vi "Draw Robot.vi"(7 "Gyro":dbl=-0.11, 8 "Starting Location":u16(ring)=2 items=["Left", "Center", "Right"], 10 "XY":cluster{"X":dbl, "Y":dbl}) -> (2 "Graph 2":cluster{cluster{"X":dbl, "Y":dbl}[]}[](graph)=[{[{"X"=44.0, "Y"=76.0}, {"X"=44.0, "Y"=76.0}]}, {[{"X"=30.03458329904793, "Y"=57.973155118857626}, {"X"=30.03458329904793, "Y"=57.973155118857626}]}, {[{"X"=29.965468303127132, "Y"=93.97308877320398}, {"X"=29.965468303127132, "Y"=93.97308877320398}]}, {[{"X"=57.96541670095207, "Y"=94.02684488114238}, {"X"=57.96541670095207, "Y"=94.02684488114238}]}, {[{"X"=58.03453169687287, "Y"=58.026911226796024}, {"X"=58.03453169687287, "Y"=58.026911226796024}]}, {[{"X"=43.942404170066, "Y"=105.9999447119553}, {"X"=43.942404170066, "Y"=105.9999447119553}]}])   [LabVIEW 2018]
panel:
  in  "Robot Lenght":dbl=44.0
  in  "Robot Width":dbl=28.0
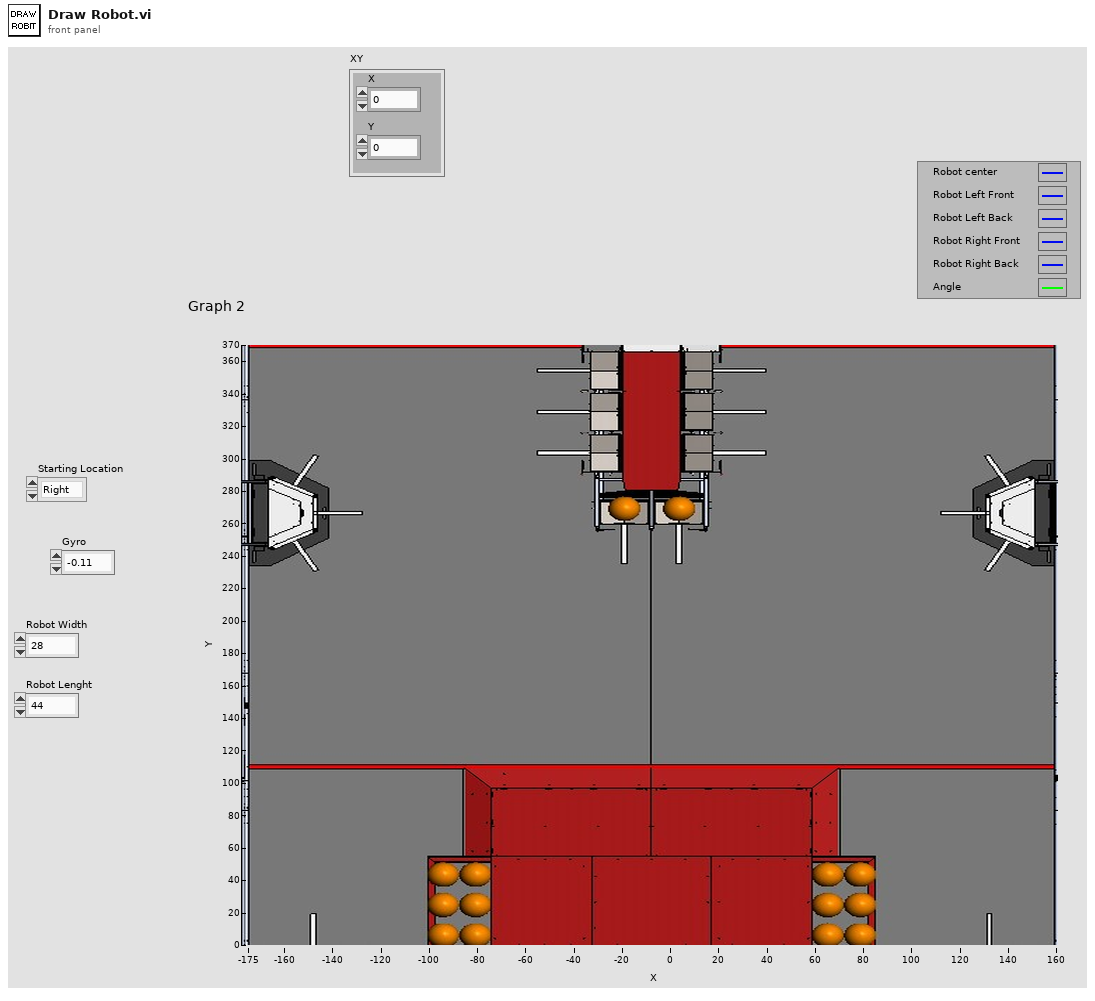
[diagram p1: front panel]
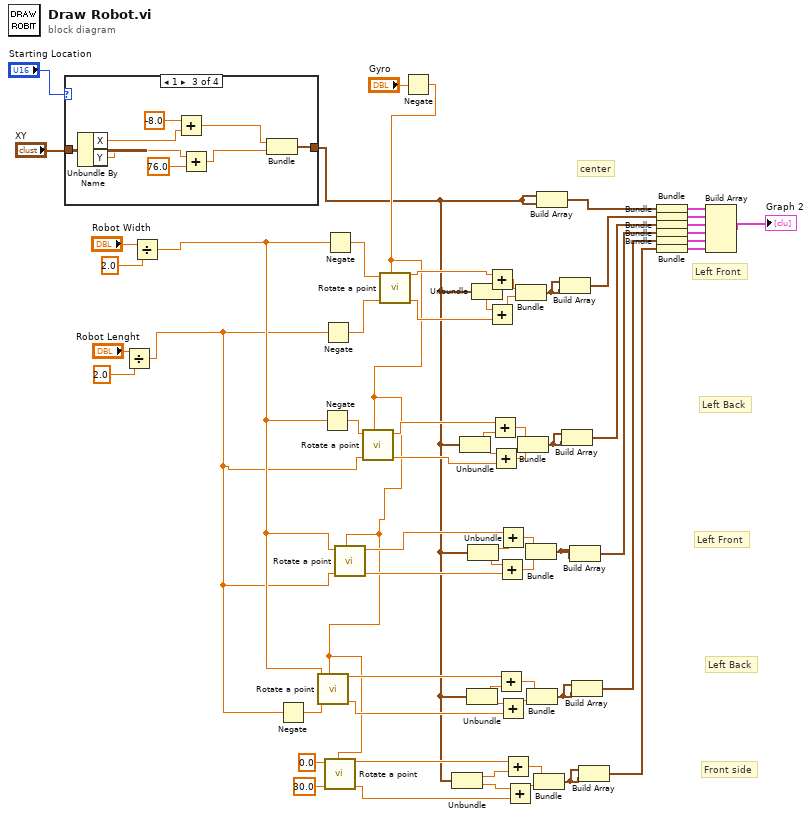
[diagram p0: block diagram]
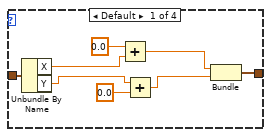
[diagram p2: hidden frame]
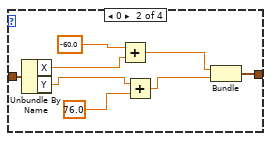
[diagram p3: hidden frame]
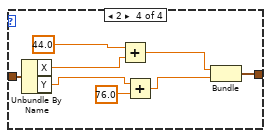
[diagram p4: hidden frame]
diagram:
  # "center"
  # "Front side"
  # "Left Back"
  # "Left Front"
  # "Left Back"
  # "Left Front"
  n1 = case shown="1" "Starting Location" {
    tunnel: "XY" -> [w73 w81 w89 w97]
    tunnel: [w72 w80 w88 w96] -> w2
    frame Default {
      n2 = Unbundle By Name(w73) -> ("X"=w71:dbl, "Y"=w69:dbl)
      n3 = Add(x=0.0, y=w71) -> (x+y=w70:dbl)
      n4 = Add(x=w69, y=0.0) -> (x+y=w68:dbl)
      n5 = Bundle(w70, w68) -> (w72:cluster{dbl, dbl})  [unwired: 1 in]
    }
    frame 0 {
      n6 = Unbundle By Name(w81) -> ("X"=w79:dbl, "Y"=w77:dbl)
      n7 = Add(x=-60.0, y=w79) -> (x+y=w78:dbl)
      n8 = Add(x=w77, y=76.0) -> (x+y=w76:dbl)
      n9 = Bundle(w78, w76) -> (w80:cluster{dbl, dbl})  [unwired: 1 in]
    }
    frame 1 {
      n10 = Unbundle By Name(w89) -> ("X"=w87:dbl, "Y"=w85:dbl)
      n11 = Add(x=-8.0, y=w87) -> (x+y=w86:dbl)
      n12 = Add(x=w85, y=76.0) -> (x+y=w84:dbl)
      n13 = Bundle(w86, w84) -> (w88:cluster{dbl, dbl})  [unwired: 1 in]
    }
    frame 2 {
      n14 = Unbundle By Name(w97) -> ("X"=w95:dbl, "Y"=w93:dbl)
      n15 = Add(x=44.0, y=w95) -> (x+y=w94:dbl)
      n16 = Add(x=w93, y=76.0) -> (x+y=w92:dbl)
      n17 = Bundle(w94, w92) -> (w96:cluster{dbl, dbl})  [unwired: 1 in]
    }
  }
  n18 = Divide(x="Robot Lenght", y=2.0) -> (x/y=w45:dbl)
  n19 = Divide(x="Robot Width", y=2.0) -> (x/y=w46:dbl)
  n20 = Negate(x=w45) -> (-x=w50:dbl)
  n21 = Negate(x=w46) -> (-x=w47:dbl)
  n22 = Negate(x=w45) -> (-x=w48:dbl)
  n23 = Negate(x=w46) -> (-x=w49:dbl)
  n24 = Negate(x="Gyro") -> (-x=w4:dbl)
  n25 = call "Rotate a point.vi"("Gyro"=w4, "Y"=w50, "X"=w46) -> ("Y'"=w21:dbl, "X'"=w22:dbl)  [unwired: 7 in]
  n26 = call "Rotate a point.vi"("Gyro"=w4, "Y"=30.0, "X"=0.0) -> ("Y'"=w16:dbl, "X'"=w15:dbl)  [unwired: 7 in]
  n27 = call "Rotate a point.vi"("Gyro"=w4, "Y"=w45, "X"=w46) -> ("Y'"=w23:dbl, "X'"=w24:dbl)  [unwired: 7 in]
  n28 = call "Rotate a point.vi"("Gyro"=w4, "Y"=w45, "X"=w47) -> ("Y'"=w33:dbl, "X'"=w34:dbl)  [unwired: 7 in]
  n29 = call "Rotate a point.vi"("Gyro"=w4, "Y"=w48, "X"=w49) -> ("Y'"=w39:dbl, "X'"=w40:dbl)  [unwired: 7 in]
  n30 = Unbundle(w2) -> (w9:dbl, w8:dbl)
  n31 = Unbundle(w2) -> (w37:dbl, w36:dbl)
  n32 = Unbundle(w2) -> (w27:dbl, w25:dbl)
  n33 = Unbundle(w2) -> (w32:dbl, w29:dbl)
  n34 = Unbundle(w2) -> (w44:dbl, w43:dbl)
  n35 = Add(x=w40, y=w44) -> (x+y=w41:dbl)
  n36 = Add(x=w43, y=w39) -> (x+y=w42:dbl)
  n37 = Add(x=w34, y=w37) -> (x+y=w38:dbl)
  n38 = Add(x=w36, y=w33) -> (x+y=w35:dbl)
  n39 = Add(x=w22, y=w27) -> (x+y=w28:dbl)
  n40 = Add(x=w29, y=w23) -> (x+y=w31:dbl)
  n41 = Add(x=w24, y=w32) -> (x+y=w30:dbl)
  n42 = Add(x=w25, y=w21) -> (x+y=w26:dbl)
  n43 = Add(x=w15, y=w9) -> (x+y=w13:dbl)
  n44 = Add(x=w8, y=w16) -> (x+y=w14:dbl)
  n45 = Bundle(w41, w42) -> (w62:cluster{dbl, dbl})  [unwired: 1 in]
  n46 = Bundle(w38, w35) -> (w61:cluster{dbl, dbl})  [unwired: 1 in]
  n47 = Bundle(w30, w31) -> (w58:cluster{dbl, dbl})  [unwired: 1 in]
  n48 = Bundle(w28, w26) -> (w59:cluster{dbl, dbl})  [unwired: 1 in]
  n49 = Bundle(w13, w14) -> (w12:cluster{dbl, dbl})  [unwired: 1 in]
  n50 = Build Array(w2, w2) -> (w64:cluster{dbl, dbl}[])
  n51 = Build Array(w62, w62) -> (w63:cluster{dbl, dbl}[])
  n52 = Build Array(w61, w61) -> (w60:cluster{dbl, dbl}[])
  n53 = Build Array(w58, w58) -> (w57:cluster{dbl, dbl}[])
  n54 = Build Array(w59, w59) -> (w56:cluster{dbl, dbl}[])
  n55 = Build Array(w12, w12) -> (w10:cluster{dbl, dbl}[])
  n56 = Bundle(w64) -> (w65:cluster{cluster{dbl, dbl}[]})  [unwired: 1 in]
  n57 = Bundle(w63) -> (w20:cluster{cluster{dbl, dbl}[]})  [unwired: 1 in]
  n58 = Bundle(w60) -> (w19:cluster{cluster{dbl, dbl}[]})  [unwired: 1 in]
  n59 = Bundle(w57) -> (w18:cluster{cluster{dbl, dbl}[]})  [unwired: 1 in]
  n60 = Bundle(w56) -> (w17:cluster{cluster{dbl, dbl}[]})  [unwired: 1 in]
  n61 = Bundle(w10) -> (w11:cluster{cluster{dbl, dbl}[]})  [unwired: 1 in]
  n62 = Build Array(w65, w20, w19, w18, w17, w11) -> (→"Graph 2":cluster{cluster{dbl, dbl}[]}[])
